vi "GetText.vi"(8 "error in":errorcluster, 11 "Shared Library Module editor node in":refnum<class "Shared Library Module editor node.lvclass">) -> (0 "error out":errorcluster, 1 "additional text":string, 2 "text":string, 3 "Shared Library Module editor node out":refnum<class "Shared Library Module editor node.lvclass">, 4 "glyph":string)   [LabVIEW 2013, in "Shared Library Module editor node.lvclass"]
doc: "Platypus Framework 1.0.1.60\nNI Systems Engineering - National Instruments"
uses:
  Shared Library Module editor node.lvclass
  <vilib>/NI/Tag Bus Data Framework/Configuration Editor/Classes/Module editor node/module editor node.lvclass
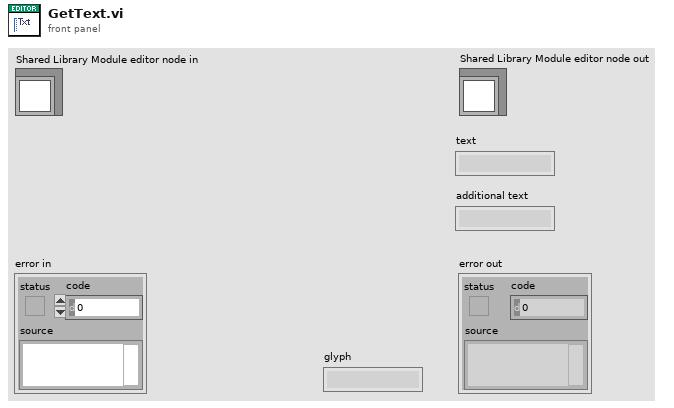
[diagram p1: front panel]
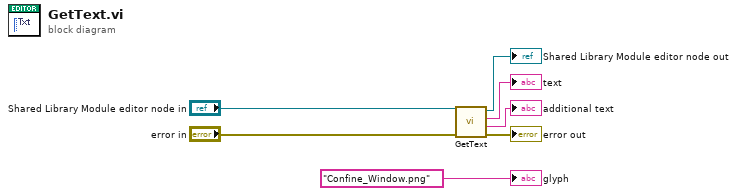
[diagram p0: block diagram]
diagram:
  n1 = call-parent "GetText.vi"("error in"="error in", "Module Editor Node in"="Shared Library Module editor node in") -> ("error out"=→"error out":errorcluster, "additional text"=→"additional text":string, "text"=→"text":string, "Module Editor Node out"=→"Shared Library Module editor node out":refnum<class "Shared Library Module editor node.lvclass">)  [unwired: 5 in, 1 out]
  "glyph" <- "Confine_Window.png" ("glyph")
